vi "RC_Client Client.vi"(8 "error in (no error)":errorcluster, 11 "RC Type":T1) -> (0 "error out":errorcluster)   [LabVIEW 2019, in "RemoteControl.lvclass"]
uses:
  RemoteControl.lvclass
  Typedefs/RC Com Type--enum.ctl
  db51367f-c7f3-480a-b132-7f33093295d6.vi
  d8d5aeaf-e1b8-48f3-8146-827dda1e4654.vi
  db51367f-c7f3-480a-b132-7f33093295d6.vi/768e530a-bae5-4f74-b090-cc074e71aae2.vi
  d8d5aeaf-e1b8-48f3-8146-827dda1e4654.vi/d22518c2-3c1a-4160-a5a9-99fc811e7fba.vi
  <vilib>/Utility/LVClass/Get LV Class Name.vi
  <vilib>/JDP Science/JSONtext/JSON text to Variant.vi
  <vilib>/JDP Science/JSONtext/LVClass Serializer/JSONtext LVClass Serializer.lvclass
panel:
  in  "milliseconds to wait":u32
  out "time (1 message) (ms)":u32
  out "messsages/s":dbl
  in  "remote port":u16=6341
  in  "address":string
  out "Parse Response":string
  out "Messages":i32
  in  "Stop":bool
  out "Command reponse":string
  out "Command":string
  out "commands":string[](array[string])
  # "CLIENT (API)"
  # "Connection info"
  # "Message Sent"
  # "Message Received"
  # "Metrics"
  # "client 1"
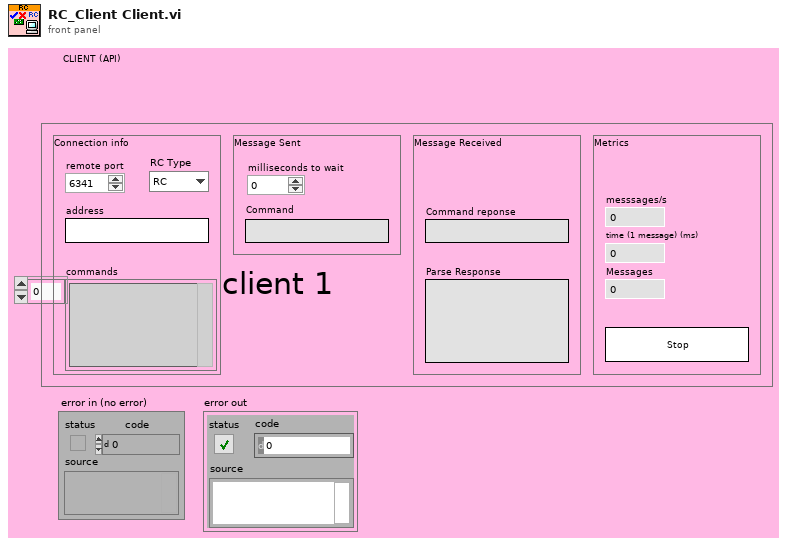
[diagram p1: front panel]
types:
  T1 = typedef "RemoteControl.lvclass/RC Com Type--enum.ctl" = enum16{"RC", "STM", "ZMQ"}
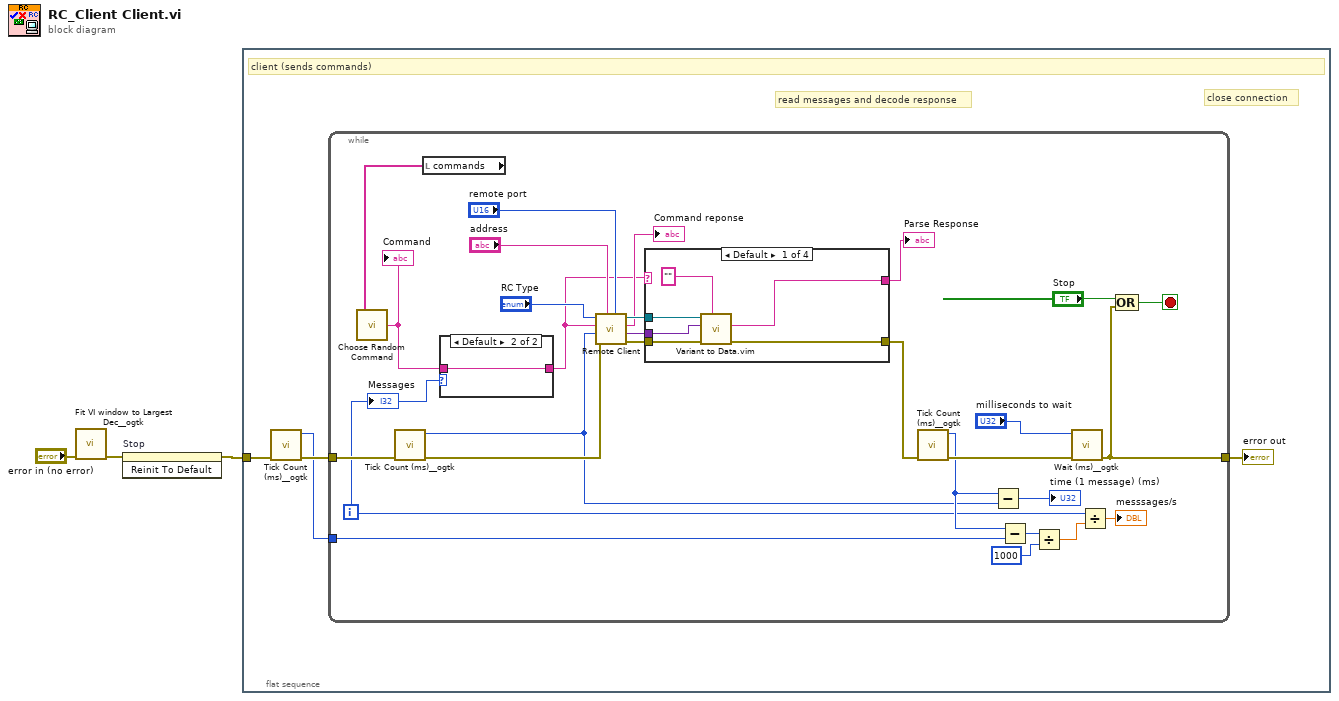
[diagram p0: block diagram]
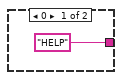
[diagram p2: hidden frame]
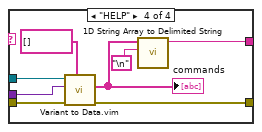
[diagram p5: hidden frame]
diagram:
  n1 = call <userlib>:"Fit VI window to Largest Dec__ogtk.vi"("error in (no error)"="error in (no error)") -> ("error out"=w3:errorcluster)  [unwired: 5 in, 1 out]
  n2 = invoke on="Stop" class="Bool" method="Reinit To Default"(error in=w3) -> (error out=w2:errorcluster)  [unwired: 2 in, 2 out]
  n3 = flat-sequence {
    tunnel: w2 -> [w4]
    frame #0 {
      # "close connection"
      # "read messages and decode response"
      # "client (sends commands)"
      n4 = call <userlib>:"Tick Count (ms)__ogtk.vi"("error in (no error)"=w4) -> ("error out"=w7:errorcluster, "millisecond timer value"=w6:u32)  [unwired: 9 in]
      n5 = while {
        tunnel: [w29] -> w5
        tunnel: w7 -> [w32]
        tunnel: w6 -> [w24]
        i -> [w16]
        stop <- w35 stop-if-true
        n6 = call <userlib>:"Tick Count (ms)__ogtk.vi"("error in (no error)"=w32) -> ("error out"=w20:errorcluster, "millisecond timer value"=w8:u32)  [unwired: 9 in]
        n7 = local read "commands"() -> (w12:string[])
        n8 = call "Choose Random Command.vi"("Array"=w12) -> ("String"=w11:string)
        "Command" <- w11
        n9 = case shown="Default" w16 {
          tunnel: ["HELP" ("Command") w37] -> w9
          tunnel: w11 -> [_ w37]
          frame 0 {
          }
          frame Default {
          }
        }
        n10 = call "Remote Client.vi"("Port"="remote port", "address"="address", "error in (no error)"=w20, "Data"=w8, "Command"=w9, "RC Type"="RC Type") -> ("error out"=w19:errorcluster, "Data out"=w21:variant, "Command out"=→"Command reponse":string, "RemoteControl out"=w23:refnum<class "RemoteControl.lvclass">)  [unwired: 2 in]
        n11 = case shown="Default" w9 {
          selector: w9 -> [_ w44 w46 _]
          tunnel: [w42 w44 w46 w49] -> w18
          tunnel: w23 -> [w41 _ _ w54]
          tunnel: w21 -> [w40 _ _ w53]
          tunnel: [w39 w45 w47 w50] -> w17
          tunnel: w19 -> [w38 w45 w47 w51]
          frame Default {
            n12 = call "Variant to Data.vim"("Data Type"="", "error in (no error)"=w38, "Data in"=w40, "RemoteControl in"=w41) -> ("error out"=w39:errorcluster, "Data out"=w42:string)  [unwired: 5 in, 1 out]
          }
          frame "open" {
          }
          frame "close" {
          }
          frame "HELP" {
            n13 = call "Variant to Data.vim"("Data Type"=string[] [], "error in (no error)"=w51, "Data in"=w53, "RemoteControl in"=w54) -> ("error out"=w50:errorcluster, "Data out"=w48:string[])  [unwired: 5 in, 1 out]
            "commands" <- w48
            n14 = call <vilib>:"1D String Array to Delimited String.vi"("delimiter"="\n", "string array"=w48) -> ("delimited string"=w49:string)  [unwired: 9 in]
          }
        }
        "Parse Response" <- w18
        n15 = call <userlib>:"Tick Count (ms)__ogtk.vi"("error in (no error)"=w17) -> ("error out"=w31:errorcluster, "millisecond timer value"=w26:u32)  [unwired: 9 in]
        n16 = Subtract(x=w26, y=w8) -> (x-y=→"time (1 message) (ms)":u32)
        n17 = Subtract(x=w26, y=w24) -> (x-y=w25:u32)
        n18 = Divide(x=w25, y=u32 1000) -> (x/y=w34:dbl)
        n19 = call <userlib>:"Wait (ms)__ogtk.vi"("error in (no error)"=w31, "milliseconds to wait"="milliseconds to wait") -> ("error out"=w29:errorcluster)  [unwired: 8 in, 1 out]
        n20 = Divide(x=w16, y=w34) -> (x/y=→"messsages/s":dbl)
        n21 = Compound Arithmetic op=OR("Stop", w29) -> (w35:bool)
        "Messages" <- w16
      }
      "error out" <- w5
    }
  }
